vi "Global_FlyWheelRPM.vi"() -> ()   [LabVIEW 2017]
panel:
  in  "Fly Wheel RPM":dbl
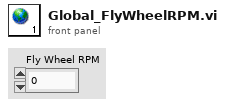
[diagram p1: front panel]
diagram:
